vi "Send Stop Polling.vi"(8 "error in (no error)":errorcluster, 11 "Message Queue in":refnum<queue>) -> (0 "error out":errorcluster, 3 "Message Queue out":refnum<queue>)   [LabVIEW 2024, in "OOQMH.lvlib" / "Stop Polling.lvclass"]
uses:
  Stop Polling.lvclass
  Stop Polling.lvclass/Stop Polling.ctl
  Message/Message.lvclass
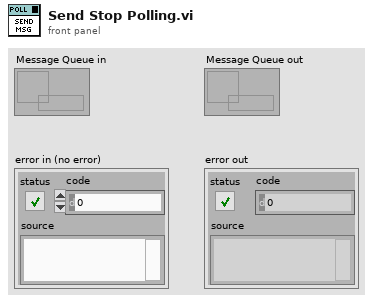
[diagram p1: front panel]
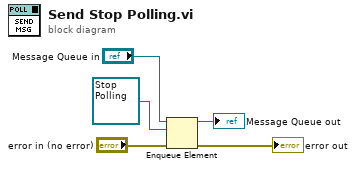
[diagram p0: block diagram]
diagram:
  n1 = Enqueue Element(queue="Message Queue in", element=refnum<class "Stop Polling.lvclass"> refnum ("OOQMH.lvlib:Stop Polling.lvclass"), error in (no error)="error in (no error)") -> (queue out=→"Message Queue out":refnum<queue>, error out=→"error out":errorcluster)  [unwired: 1 in, 1 out]
